vi "test_char_to_float.vi"() -> ()   [LabVIEW 2020]
panel:
  out "*(type *) &x 6":dbl
  in  "index 2":i32
  in  "data out 2":string
  out "*(type *) &x 5":sgl
  in  "Float 2":sgl=12.961126 format="%#_8g"
  out "*(type *) &x 4":sgl
  out "hex integer string":string[](array[string])=["41", "4F", "60", "C6"]
  out "*(type *) &x 3":u8[](array[numeric])=[65, 79, 96, 198] format="%.0x"
  in  "Float":sgl=12.961126 format="%#_8g"
  out "appended array":u8[](array[numeric])
  out "*(type *) &x 2":dbl
  out "lo(x) 2":u8
  out "hi(x) 2":u8
  out "lo(x)":u8
  out "hi(x)":u8
  out "*(type *) &x":dbl
  out "number 3":dbl
  out "string":string
  out "number 2":dbl
  out "number":dbl
  out "single precision float":sgl[](array[numeric])
  out "deleted portion":u8[](array[numeric]) format="%x"
  in  "index":i32
  in  "data out":string
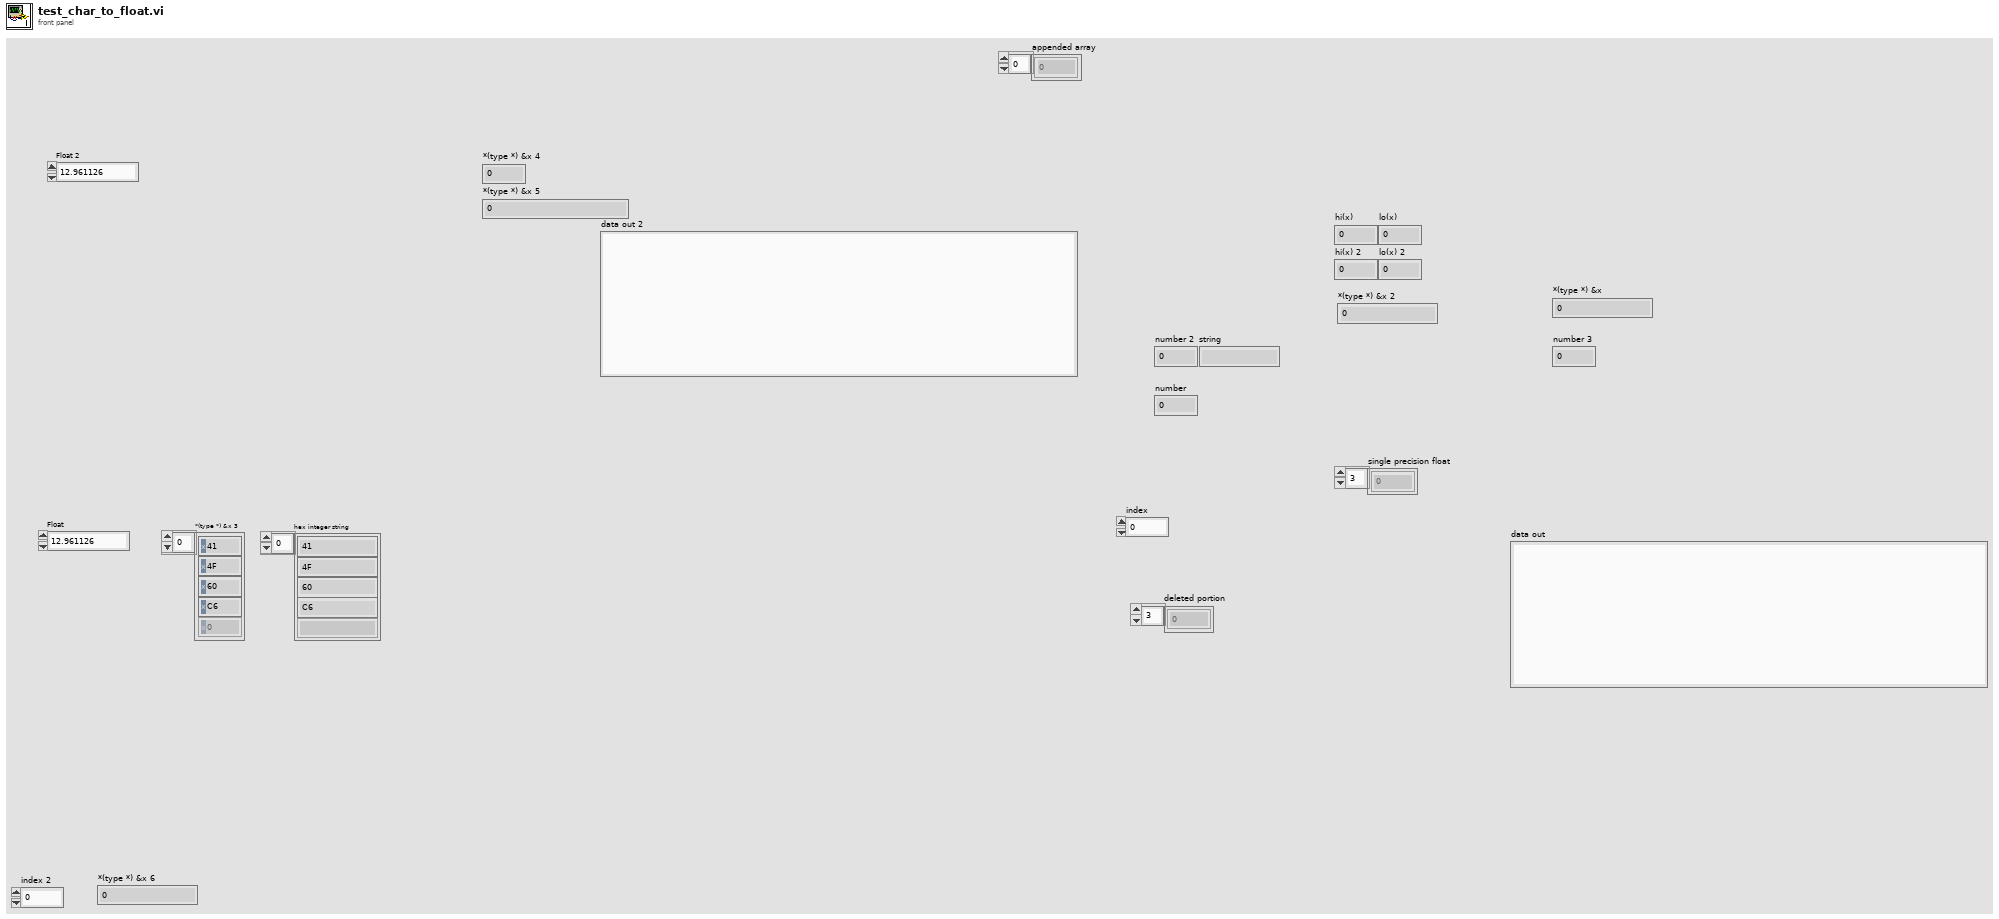
[diagram p1: front panel]
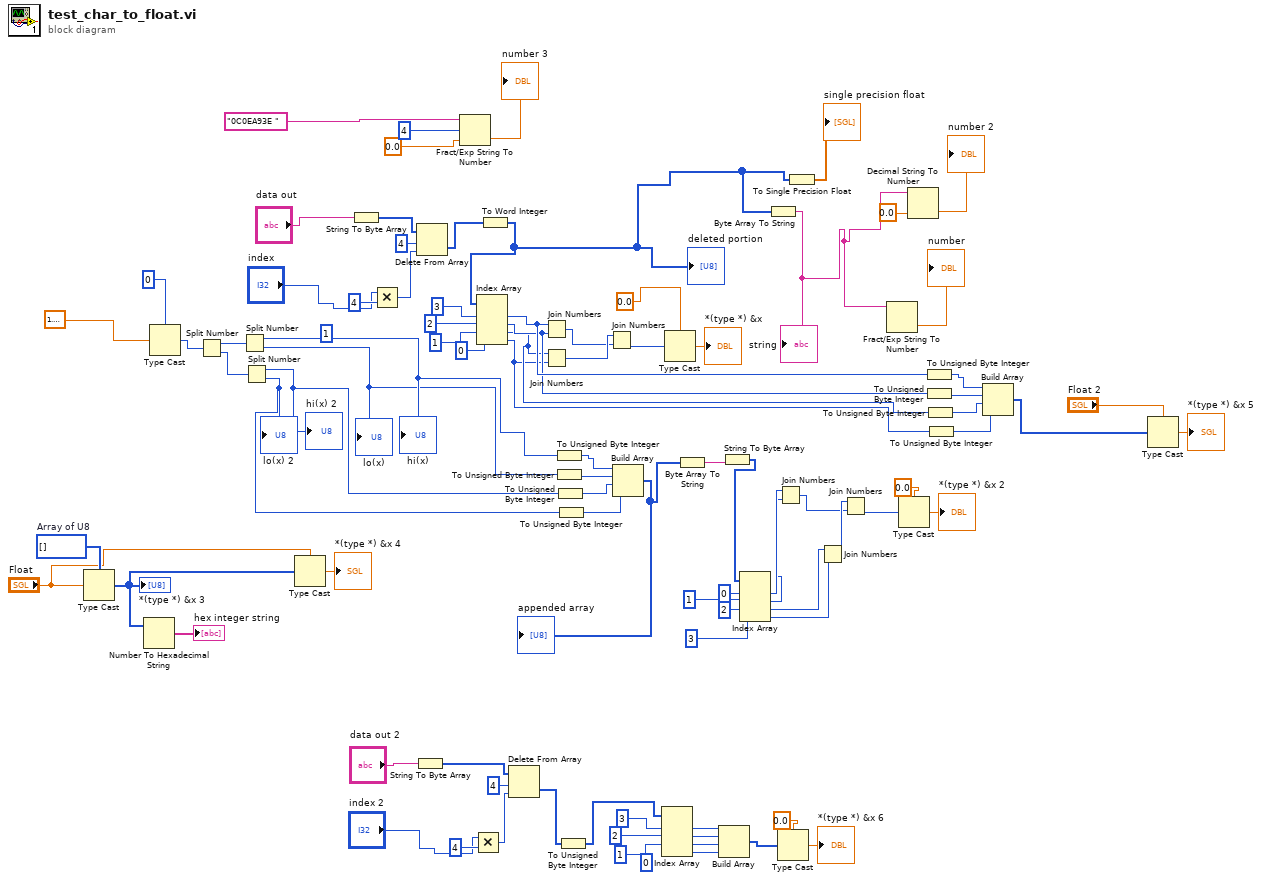
[diagram p0: block diagram]
diagram:
  (unwired) 0 ("index")
  w36 = u8[] []  # Array of U8
  (unwired) 1 ("y")
  n1 = Type Cast(type=w36, x="Float") -> (*(type *) &x=w34:u8[])
  "*(type *) &x 3" <- w34
  n2 = Number To Hexadecimal String(2:w34) -> (0:→"hex integer string":string[])  [unwired: 1 in]
  n3 = Type Cast(type=0 ("index"), x=sgl 1.7 ("number")) -> (*(type *) &x=w63:i32)
  n4 = Split Number(x=w63) -> (hi(x)=w62:u16, lo(x)=w61:u16)
  n5 = Split Number(x=w62) -> (hi(x)=w55:u8, lo(x)=w54:u8)
  "hi(x)" <- w55
  "lo(x)" <- w54
  n6 = Split Number(x=w61) -> (hi(x)=w53:u8, lo(x)=w52:u8)
  "hi(x) 2" <- w53
  "lo(x) 2" <- w52
  n7 = Type Cast(type="Float", x=w34) -> (*(type *) &x=→"*(type *) &x 4":sgl)
  n8 = String To Byte Array(string="data out") -> (unsigned byte array=w88:u8[])
  n9 = Multiply(x="index", y=4) -> (x*y=w86:i32)
  n10 = String To Byte Array(string="data out 2") -> (unsigned byte array=w15:u8[])
  n11 = Delete From Array(array=w88, length=4, index=w86) -> (deleted portion=w75:u8[])  [unwired: 1 out]
  n12 = Fract/Exp String To Number(string="0C0EA93E ", offset=4, default (0 dbl)=0.0 ("number 2")) -> (number=→"number 3":dbl)  [unwired: 1 in, 1 out]
  n13 = Multiply(x="index 2", y=4) -> (x*y=w14:i32)
  n14 = To Word Integer(number=w75) -> (16bit integer=w31:i16[])
  "deleted portion" <- w31
  n15 = Index Array(array=w31, index #1=3 ("index"), index #2=2 ("index"), index #3=1 ("index"), index #4=0 ("index")) -> (element #1=w23:i16, element #2=w22:i16, element #3=w21:i16, element #4=w20:i16)
  n16 = Delete From Array(array=w15, length=4, index=w14) -> (deleted portion=w12:u8[])  [unwired: 1 out]
  n17 = Join Numbers(hi=w23, lo=w22) -> ((hi.lo)=w66:u32)
  n18 = Join Numbers(hi=w21, lo=w20) -> ((hi.lo)=w67:u32)
  n19 = To Unsigned Byte Integer(number=w55) -> (unsigned 8bit integer=w50:u8)
  n20 = To Unsigned Byte Integer(number=w54) -> (unsigned 8bit integer=w51:u8)
  n21 = To Unsigned Byte Integer(number=w53) -> (unsigned 8bit integer=w49:u8)
  n22 = To Unsigned Byte Integer(number=w52) -> (unsigned 8bit integer=w48:u8)
  n23 = To Unsigned Byte Integer(number=w12) -> (unsigned 8bit integer=w8:u8[])
  n24 = Join Numbers(hi=w67, lo=w66) -> ((hi.lo)=w70:u64)
  n25 = Build Array(w50, w51, w49, w48) -> (w38:u8[])
  "appended array" <- w38
  n26 = Index Array(array=w8, index #1=3 ("index"), index #2=2 ("index"), index #3=1 ("index")) -> (element #1=w7:u8, element #2=w6:u8, element #3=w5:u8, element #4=w4:u8)  [unwired: 1 in]
  n27 = Type Cast(type=sgl 0.0 ("number"), x=w70) -> (*(type *) &x=→"*(type *) &x":sgl)
  n28 = Byte Array To String(unsigned byte array=w38) -> (string=w37:string)
  n29 = Build Array(w7, w6, w5, w4) -> (w1:u8[])
  n30 = String To Byte Array(string=w37) -> (unsigned byte array=w28:u8[])
  n31 = Index Array(array=w28, index #1=0 ("index"), index #2=1 ("index"), index #3=2 ("index"), index #4=3 ("index")) -> (element #1=w43:u8, element #2=w42:u8, element #3=w41:u8, element #4=w40:u8)
  n32 = Byte Array To String(unsigned byte array=w31) -> (string=w82:string)
  "string" <- w82
  n33 = Join Numbers(hi=w43, lo=w42) -> ((hi.lo)=w57:u16)
  n34 = Type Cast(type=sgl 0.0 ("number"), x=w1) -> (*(type *) &x=→"*(type *) &x 6":sgl)
  n35 = To Single Precision Float(number=w31) -> (single precision float=→"single precision float":sgl[])
  n36 = Join Numbers(hi=w41, lo=w40) -> ((hi.lo)=w58:u16)
  n37 = Join Numbers(hi=w58, lo=w57) -> ((hi.lo)=w60:u32)
  n38 = Fract/Exp String To Number(string=w82) -> (number=→"number":dbl)  [unwired: 3 in, 1 out]
  n39 = Type Cast(type=sgl 0.0 ("number"), x=w60) -> (*(type *) &x=→"*(type *) &x 2":sgl)
  n40 = Decimal String To Number(string=w82, default (0L)=0.0 ("default (0 I32)")) -> (number=→"number 2":dbl)  [unwired: 1 in, 1 out]
  n41 = To Unsigned Byte Integer(number=w23) -> (unsigned 8bit integer=w26:u8)
  n42 = To Unsigned Byte Integer(number=w22) -> (unsigned 8bit integer=w27:u8)
  n43 = To Unsigned Byte Integer(number=w21) -> (unsigned 8bit integer=w25:u8)
  n44 = To Unsigned Byte Integer(number=w20) -> (unsigned 8bit integer=w24:u8)
  n45 = Build Array(w26, w27, w25, w24) -> (w19:u8[])
  n46 = Type Cast(type="Float 2", x=w19) -> (*(type *) &x=→"*(type *) &x 5":sgl)
